vi "AlliGator Draw Phasor Plot UC.vi"(7 "# Ticks":i32=11, 8 "Error In":errorcluster, 11 "Phasor Plot Image  in":T2) -> (0 "Error Out":errorcluster, 1 "Font, Size & Style":T1, 2 "Phasor Plot Frame Reference Points":T3, 3 "Phasor Plot Image out":T2)   [LabVIEW 2021, in "AlliGator Phasor Plot.lvlib"]
doc: "Draws the UC in the Phasor Plot image."
uses:
  AlliGator Phasor Plot.lvlib
  <vilib>/vision/Image Controls.llb/IMAQ Image.ctl
  Phasor Ratio/AlliGator Phasor Plot Reference Points.ctl
  Phasor/Phasor SEPL Tick Data.ctl
  Phasor/Phasor (g, s).ctl
  Phasor Ratio/AlliGator Phasor Ratio.lvlib
  Utilities/Utilities.lvlib
  Math/Math.lvlib
  Settings/AlliGator Settings.lvlib
  Phasor/Phasor.lvlib
panel:
  # "see the AlliGator License on the block diagram (Ctrl+E or Window:Show Block Diagram)"
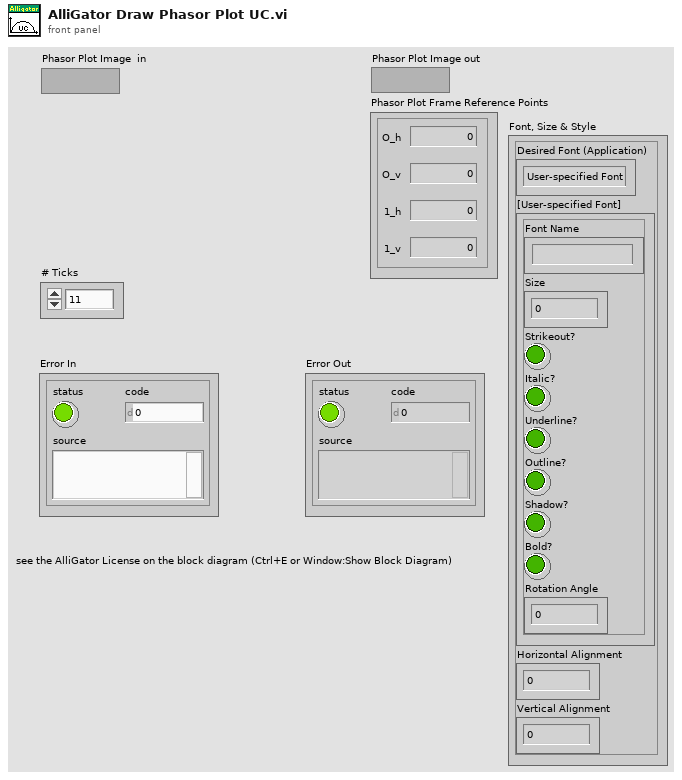
[diagram p1: front panel]
types:
  T1 = cluster{"Desired Font (Application)":enum16{"User-specified Font", "Application Font", "System Font", "Dialog Font"}, "[User-specified Font]":cluster{"Font Name":string, "Size":i16, "Strikeout?":bool, "Italic?":bool, "Underline?":bool, "Outline?":bool, "Shadow?":bool, "Bold?":bool, "Rotation Angle":dbl}, "Horizontal Alignment":i16, "Vertical Alignment":i16}
  T2 = typedef "IMAQ Image.ctl" = refnum<image>
  T3 = typedef "AlliGator Phasor Ratio.lvlib/AlliGator Phasor Plot Reference Points.ctl" = cluster{"O_h":dbl, "O_v":dbl, "1_h":dbl, "1_v":dbl}
  T4 = typedef "AlliGator Settings.lvlib/AlliGator Phasor Plot Graphics Options.ctl" = cluster{"UC Color":u32, "Show UC Tau Ticks":bool, "SEPL Color":u32, "Show SEPL Tau Ticks":bool, "Axes Color":u32, "Show (g,s) Ticks":bool, "Show UC":bool, "Show SEPL":bool, "Show Axes":bool, "Show UC Tau Labels":bool, "Show SEPL Tau Labels":bool, "Show (g,s) Labels":bool, "UC Label Size":i16, "UC Label Distance":dbl, "SEPL Label Size":i16, "SEPL Label Distance":dbl, "Axes Label Size":i16, "Axes Label Distance":dbl}
  T5 = typedef "AlliGator Phasor Plot.lvlib/AlliGator Phasor Plot Size.ctl" = cluster{"H":i32, "V":i32, "Margin":dbl}
  T6 = cluster{"UCl":dbl, "UCt":dbl, "UCr":dbl, "UCb":dbl}
  T7 = typedef "Phasor.lvlib/Phasor SEPL Tick Data.ctl" = cluster{"tau_i (ns)":dbl, "Tick start (g, s)":T8, "Tick (dg, ds)":T8, "long tick?":bool}
  T8 = typedef "Phasor.lvlib/Phasor (g, s).ctl" = cluster{"g":dbl, "s":dbl}
  T9 = cluster{"Phasor Plot x":dbl, "Phasor Plot y":dbl}
  T10 = typedef "Utilities.lvlib/For Loop Iteration Type.ctl" = enum16{"default", "first", "last", "out of range"}
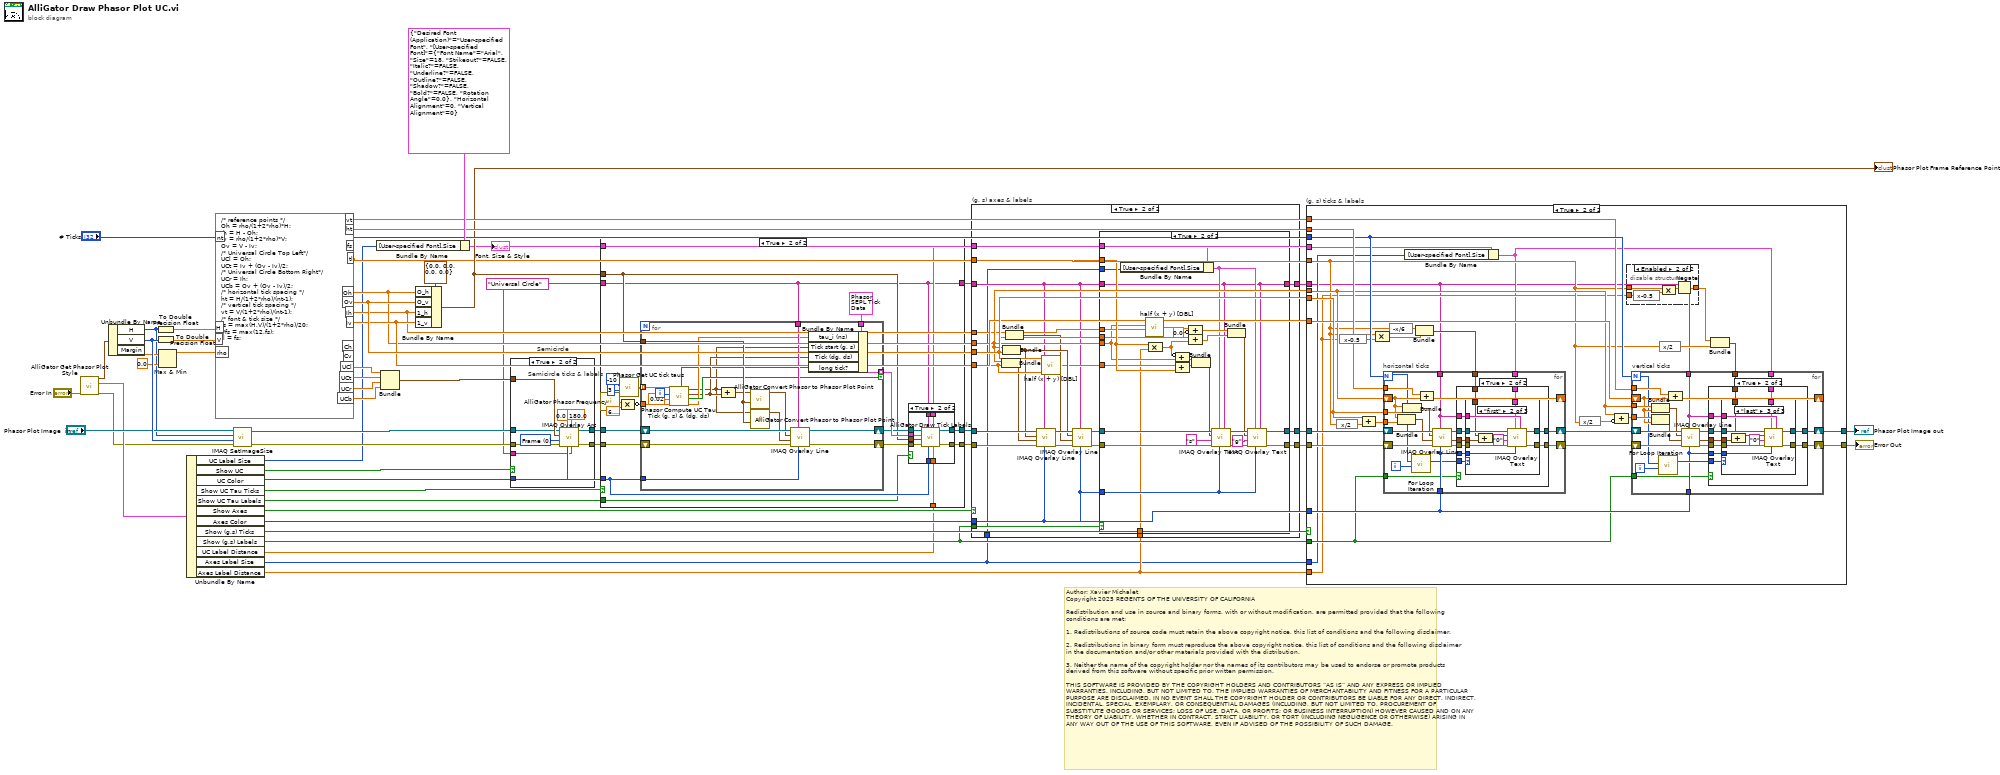
[diagram p0: block diagram]
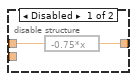
[diagram p7: hidden frame]
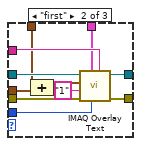
[diagram p10: hidden frame]
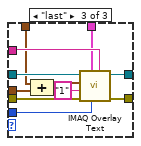
[diagram p13: hidden frame]
diagram:
  w13 = "Universal Circle" ("Group")
  # "Author: Xavier Michalet\nCopyright 2025 REGENTS OF THE UNIVERSITY OF CALIFORNIA\n\nRedistribution and use in source and binary forms, with or without modification, are permitted provided that the following conditions are met:\n\n1. Redistributions of source code must retain the above copyright notice, this list of conditions and the following disclaimer.\n\n2. Redistributions in binary form must reproduce the above copyright notice, this list of conditions and the following disclaimer in the documentation and/or other materials provided with the distribution.\n\n3. Neither the name of the copyright holder nor the names of its contributors may be used to endorse or promote products derived from this software without specific prior written permission.\n\nTHIS SOFTWARE IS PROVIDED BY THE COPYRIGHT HOLDERS AND CONTRIBUTORS “AS IS” AND ANY EXPRESS OR IMPLIED WARRANTIES, INCLUDING, BUT NOT LIMITED TO, THE IMPLIED WARRANTIES OF MERCHANTABILITY AND FITNESS FOR A PARTICULAR PURPOSE ARE DISCLAIMED. IN NO EVENT SHALL THE COPYRIGHT HOLDER OR CONTRIBUTORS BE LIABLE FOR ANY DIRECT, INDIRECT, INCIDENTAL, SPECIAL, EXEMPLARY, OR CONSEQUENTIAL DAMAGES (INCLUDING, BUT NOT LIMITED TO, PROCUREMENT OF SUBSTITUTE GOODS OR SERVICES; LOSS OF USE, DATA, OR PROFITS; OR BUSINESS INTERRUPTION) HOWEVER CAUSED AND ON ANY THEORY OF LIABILITY, WHETHER IN CONTRACT, STRICT LIABILITY, OR TORT (INCLUDING NEGLIGENCE OR OTHERWISE) ARISING IN ANY WAY OUT OF THE USE OF THIS SOFTWARE, EVEN IF ADVISED OF THE POSSIBILITY OF SUCH DAMAGE."
  n1 = call "AlliGator Get Phasor Plot Style.vi"("Error In"="Error In") -> ("Error Out"=w15:errorcluster, "Phasor Plot Graphics Options"=w18:T4, "Phasor Plot Size"=w17:T5)  [unwired: 8 in]
  n2 = Unbundle By Name(w17) -> ("H"=w8:i32, "V"=w45:i32, "Margin"=w37:dbl)
  n3 = To Double Precision Float(number=w8) -> (double precision float=w48:dbl)
  n4 = To Double Precision Float(number=w45) -> (double precision float=w47:dbl)
  n5 = Max & Min(x=w37, y=0.0) -> (max(x,y)=w35:dbl)  [unwired: 1 out]
  n6 = Unbundle By Name(w18) -> ("UC Label Size"=w6:i16, "Show UC"=w25:bool, "UC Color"=w23:u32, "Show UC Tau Ticks"=w24:bool, "Show UC Tau Labels"=w10:bool, "Show Axes"=w26:bool, "Axes Color"=w30:u32, "Show (g,s) Ticks"=w27:bool, "Show (g,s) Labels"=w11:bool, "UC Label Distance"=w5:dbl, "Axes Label Size"=w3:i16, "Axes Label Distance"=w4:dbl)
  n7 = formula code="/* reference points */\nOh = rho/(1+2*rho)*H;\nIh = H - Oh;\nIv = rho/(1+2*rho)*V;\nOv = V - Iv;\n/* Universal Circle Top Left*/\nUCl = Oh;\nUCt = Iv + (Ov - Iv)/2;\n/* Universal Circle Bottom Right*/\nUCr = Ih;\nUCb = Ov + (Ov - Iv)/2;\n/* horizontal tick spacing */\nht = H/(1+2*rho)/(nt-1);\n/* vertical tick spacing */\nvt = V/(1+2*rho)/(nt-1);\n/* font & tick size */\nfs = max(H,V)/(1+2*rho)/20;\n//fs = max(12,fs);\ntl = fs;"("H"=w48, "V"=w47, "rho"=w35, "nt"="# Ticks") -> ("Oh"=w32:dbl, "Ov"=w34:dbl, "Ih"=w31:dbl, "Iv"=w33:dbl, "UCl"=w51:dbl, "UCt"=w52:dbl, "UCr"=w50:dbl, "UCb"=w49:dbl, "ht"=w42:dbl, "vt"=w38:dbl, "tl"=w7:dbl)  [unwired: 3 out]
  n8 = call "IMAQ SetImageSize"("error in (no error)"=w15, "Y Resolution"=w45, "X Resolution"=w8, "Image"="Phasor Plot Image  in") -> ("error out"=w43:errorcluster, "Image Out"=w46:T2)  [unwired: 1 in]
  n9 = Bundle By Name(cluster=T1 {"Desired Font (Application)"=enum."User-specified Font", "[User-specified Font]"={"Font Name"="Arial", "Size"=18, "Strikeout?"=FALSE, "Italic?"=FALSE, "Underline?"=FALSE, "Outline?"=FALSE, "Shadow?"=FALSE, "Bold?"=FALSE, "Rotation Angle"=0.0}, "Horizontal Alignment"=0, "Vertical Alignment"=0} ("Font, Size & Style"), "[User-specified Font].Size"=w6) -> (w9:T1)
  "Font, Size & Style" <- w9
  n10 = Bundle("UCl"=w51, "UCt"=w52, "UCr"=w50, "UCb"=w49) -> (w14:T6)  [unwired: 1 in]
  n11 = Bundle By Name(cluster=T3 {"O_h"=0.0, "O_v"=0.0, "1_h"=0.0, "1_v"=0.0} ("Phasor Plot Reference Points"), "O_h"=w32, "O_v"=w34, "1_h"=w31, "1_v"=w33) -> (w12:T3)
  "Phasor Plot Frame Reference Points" <- w12
  n12 = case "Semicircle" shown="True" w25 {
    tunnel: w14 -> [_ w66]
    tunnel: w46 -> [w56 w65]
    tunnel: w43 -> [w55 w64]
    tunnel: w23 -> [_ w63]
    tunnel: [w56 w59] -> w22
    tunnel: [w55 w58] -> w21
    tunnel: w13 -> [_ w57]
    frame False {
    }
    frame True {
      w62 = u32 0 items=["Frame", "Fill"] ("Drawing Mode (Frame)")
      n13 = call "IMAQ Overlay Arc"("Group"=w57, "End Angle (degrees)"=180.0, "Color"=w63, "Start Angle (degrees)"=0.0, "error in (no error)"=w64, "Drawing Mode (Frame)"=w62, "Bounding Rectangle"=w66, "Image"=w65) -> ("error out"=w58:errorcluster, "Image Out"=w59:T2)  [unwired: 2 in]
    }
  }
  n14 = case "Semicircle ticks & labels" shown="True" w24 {
    tunnel: w23 -> [_ w76]
    tunnel: [w69 w81] -> w20
    tunnel: w22 -> [w69 w85]
    tunnel: [w68 w79] -> w19
    tunnel: w21 -> [w68 w84]
    tunnel: w13 -> [w67 w70]
    tunnel: w12 -> [_ w72]
    tunnel: w10 -> [_ w75]
    tunnel: w9 -> [_ w78]
    tunnel: w5 -> [_ w71]
    tunnel: [w67 w70] -> w2
    frame False {
    }
    frame True {
      n15 = call "AlliGator Phasor Frequency.vi"() -> ("Phasor Frequency"=w88:dbl[unit])
      n16 = call "Phasor Get UC tick taus.vi"("Log Tick Start (-10: 100 ps)"=-10, "# Decades (4: 10 ps - 900 ns)"=3) -> ("Array of taus"=w89:dbl[unit][])  [unwired: 6 in]
      n17 = Compound Arithmetic op=MULTIPLY(w88, 6.283185307179586) -> (invert w87:dbl[unit])
      n18 = for {
        tunnel: w89 -> [w122] mode=indexing
        tunnel: w87 -> [w120]
        tunnel: w72 -> [w119]
        shift-right: [w114] -> w82
        shift-left: w85 -> [w118]
        shift-right: [w113] -> w80
        shift-left: w84 -> [w115]
        tunnel: w70 -> [w112]
        tunnel: w76 -> [w111]
        tunnel: [w105] -> w83 mode=indexing if=w108
        tunnel: T7 {"tau_i (ns)"=0.0, "Tick start (g, s)"={"g"=0.0, "s"=0.0}, "Tick (dg, ds)"={"g"=0.0, "s"=0.0}, "long tick?"=FALSE} -> [w102]
        i -> [w121]
        n19 = call "Phasor Compute UC Tau Tick (g, s) & (dg, ds).vi"("1/2 pi f"=w120, "Tick Length (0.01)"=0.02, "Tick Index"=w121, "tau_i"=w122) -> ("tau_i (ns)"=w107:dbl, "label?"=w108:bool, "Tick (dg, ds)"=w106:T8, "Tick start (g, s)"=w103:T8, "long tick?"=w104:bool)  [unwired: 3 in]
        n20 = Compound Arithmetic op=ADD(w103, w106) -> (w109:T8)
        n21 = call "AlliGator Convert Phasor to Phasor Plot Point.vi"("Phasor Plot Reference Points"=w119, "Phasor"=w109) -> ("Phasor Plot Point"=w117:T9)  [unwired: 9 in]
        n22 = call "AlliGator Convert Phasor to Phasor Plot Point.vi"("Phasor Plot Reference Points"=w119, "Phasor"=w103) -> ("Phasor Plot Point"=w116:T9)  [unwired: 9 in]
        n23 = call "IMAQ Overlay Line"("Color"=w111, "Group"=w112, "error in (no error)"=w115, "End Point"=w116, "Start Point"=w117, "Image"=w118) -> ("error out"=w113:errorcluster, "Image Out"=w114:T2)  [unwired: 4 in]
        n24 = Bundle By Name(cluster=w102, "tau_i (ns)"=w107, "Tick start (g, s)"=w103, "Tick (dg, ds)"=w106, "long tick?"=w104) -> (w105:T7)
      }
      n25 = case shown="True" w75 {
        tunnel: w83 -> [_ w94]
        tunnel: w82 -> [w91 w101]
        tunnel: [w91 w100] -> w81
        tunnel: w80 -> [w90 w99]
        tunnel: [w90 w98] -> w79
        tunnel: w70 -> [_ w97]
        tunnel: w78 -> [_ w96]
        tunnel: w76 -> [_ w95]
        tunnel: w72 -> [_ w93]
        tunnel: w71 -> [_ w92]
        frame False {
        }
        frame True {
          n26 = call "AlliGator Draw Tick Labels.vi"("Label Distance (tick unit)"=w92, "Font, Size & Style"=w96, "Text Color"=w95, "Overlay Group"=w97, "error in (no error)"=w99, "Phasor Plot Reference Points"=w93, "Tick Label Data"=w94, "Refnum in"=w101) -> ("error out"=w98:errorcluster, "Refnum out"=w100:T2)  [unwired: 2 in]
        }
      }
    }
  }
  n27 = case "(g, s) axes & labels" shown="True" w26 {
    tunnel: w9 -> [_ w149]
    tunnel: w7 -> [_ w148]
    tunnel: w34 -> [_ w147]
    tunnel: w33 -> [_ w146]
    tunnel: w32 -> [_ w145]
    tunnel: w31 -> [_ w144]
    tunnel: w30 -> [_ w129]
    tunnel: w20 -> [w125 w143]
    tunnel: w19 -> [w124 w140]
    tunnel: [w125 w134] -> w29
    tunnel: [w124 w133] -> w28
    tunnel: w2 -> [w123 w131]
    tunnel: w11 -> [_ w130]
    tunnel: w3 -> [_ w128]
    tunnel: w4 -> [_ w127]
    tunnel: [w123 w126] -> w1
    frame False {
    }
    frame True {
      n28 = Bundle("Oh"=w145, "Iv"=w146) -> (w137:cluster{"Oh":dbl, "Iv":dbl})  [unwired: 1 in]
      n29 = Bundle("Oh"=w145, "Ov"=w147) -> (w136:cluster{"Oh":dbl, "Ov":dbl})  [unwired: 1 in]
      n30 = Bundle("Ih"=w144, "Ov"=w147) -> (w135:cluster{"Ih":dbl, "Ov":dbl})  [unwired: 1 in]
      n31 = call "IMAQ Overlay Line"("Color"=w129, "Group"=w131, "error in (no error)"=w140, "End Point"=w137, "Start Point"=w136, "Image"=w143) -> ("error out"=w141:errorcluster, "Image Out"=w142:T2)  [unwired: 4 in]
      n32 = call "half (x + y) [DBL].vi"("y"=w146, "x"=w147) -> ("(x+y)/2"=w132:dbl)  [unwired: 4 in]
      n33 = call "IMAQ Overlay Line"("Color"=w129, "Group"=w131, "error in (no error)"=w141, "End Point"=w135, "Start Point"=w136, "Image"=w142) -> ("error out"=w138:errorcluster, "Image Out"=w139:T2)  [unwired: 4 in]
      n34 = case shown="True" w130 {
        tunnel: w149 -> [_ w180]
        tunnel: w148 -> [_ w179]
        tunnel: w147 -> [_ w178]
        tunnel: w145 -> [_ w155]
        tunnel: w144 -> [_ w177]
        tunnel: w139 -> [w152 w176]
        tunnel: w138 -> [w151 w175]
        tunnel: [w152 w164] -> w134
        tunnel: [w151 w163] -> w133
        tunnel: w132 -> [_ w162]
        tunnel: w131 -> [w150 w153]
        tunnel: w129 -> [_ w158]
        tunnel: w128 -> [_ w156]
        tunnel: w127 -> [_ w154]
        tunnel: [w150 w153] -> w126
        frame False {
        }
        frame True {
          n35 = Bundle By Name(cluster=w180, "[User-specified Font].Size"=w156) -> (w157:T1)
          n36 = call "half (x + y) [DBL].vi"("y"=w177, "x"=w155) -> ("(x+y)/2"=w161:dbl)  [unwired: 4 in]
          n37 = Compound Arithmetic op=MULTIPLY(w179, w154) -> (w159:dbl)
          n38 = Compound Arithmetic op=ADD(invert w159, w155) -> (w170:dbl)
          n39 = Compound Arithmetic op=ADD(w162, w179) -> (w169:dbl)
          n40 = Compound Arithmetic op=ADD(w161, invert 0.0 ("value")) -> (w167:dbl)
          n41 = Compound Arithmetic op=ADD(w178, w159) -> (w166:dbl)
          n42 = Bundle(w170, w169) -> (w168:cluster{dbl, dbl})  [unwired: 1 in]
          n43 = call "IMAQ Overlay Text"("Group"=w153, "Text Color (black)"=w158, "Font, Size & Style"=w157, "error in (no error)"=w175, "String"="s", "Origin"=w168, "Image"=w176) -> ("error out"=w174:errorcluster, "Image Out"=w173:T2)  [unwired: 3 in]
          n44 = Bundle(w167, w166) -> (w165:cluster{dbl, dbl})  [unwired: 1 in]
          n45 = call "IMAQ Overlay Text"("Group"=w153, "Text Color (black)"=w158, "Font, Size & Style"=w157, "error in (no error)"=w174, "String"="g", "Origin"=w165, "Image"=w173) -> ("error out"=w163:errorcluster, "Image Out"=w164:T2)  [unwired: 3 in]
        }
      }
    }
  }
  n46 = case "(g, s) ticks & labels" shown="True" w27 {
    tunnel: w42 -> [_ w213]
    tunnel: [w182 w212] -> w41
    tunnel: [w181 w211] -> w40
    tunnel: "# Ticks" -> [_ w210]
    tunnel: w38 -> [_ w209]
    tunnel: w9 -> [_ w186]
    tunnel: w7 -> [_ w191]
    tunnel: w34 -> [_ w208]
    tunnel: w33 -> [_ w207]
    tunnel: w32 -> [_ w206]
    tunnel: w30 -> [_ w205]
    tunnel: w29 -> [w182 w204]
    tunnel: w28 -> [w181 w203]
    tunnel: w11 -> [_ w190]
    tunnel: w4 -> [_ w188]
    tunnel: w3 -> [_ w185]
    tunnel: w1 -> [_ w183]
    frame False {
    }
    frame True {
      n47 = expression code="x/2"(w191) -> (w201:dbl)
      n48 = expression code="x-0.5"(w188) -> (w184:dbl)
      n49 = Compound Arithmetic op=ADD(w208, w201) -> (w202:dbl)
      n50 = Compound Arithmetic op=MULTIPLY(w191, w184) -> (w189:dbl)
      n51 = expression code="-x/6"(w191) -> (w195:dbl)
      n52 = Bundle By Name(cluster=w186, "[User-specified Font].Size"=w185) -> (w187:T1)
      n53 = Bundle("tl"=w195, w189) -> (w196:cluster{"tl":dbl, dbl})  [unwired: 1 in]
      n54 = for "horizontal ticks" {
        N: w210 -> [w283]
        shift-right: [w288] -> w200
        shift-left: w204 -> [w298]
        shift-right: [w287] -> w199
        shift-left: w203 -> [w297]
        shift-right: [w294] -> _
        shift-left: w206 -> [w292]
        tunnel: w205 -> [w285]
        tunnel: w213 -> [w293]
        tunnel: w202 -> [w291]
        tunnel: w183 -> [w286]
        tunnel: w208 -> [w296]
        tunnel: w187 -> [w281]
        tunnel: w196 -> [w279]
        tunnel: w190 -> [w278]
        i -> [w284]
        n55 = Bundle("Oh"=w292, w291) -> (w280:cluster{"Oh":dbl, dbl})  [unwired: 1 in]
        n56 = Bundle("Oh"=w292, "Ov"=w296) -> (w295:cluster{"Oh":dbl, "Ov":dbl})  [unwired: 1 in]
        n57 = call "For Loop Iteration.vi"("i"=w284, "N"=w283) -> ("Iteration"=w282:T10)  [unwired: 8 in, 1 out]
        n58 = Compound Arithmetic op=ADD(w293, w292) -> (w294:dbl)
        n59 = call "IMAQ Overlay Line"("Color"=w285, "Group"=w286, "error in (no error)"=w297, "End Point"=w280, "Start Point"=w295, "Image"=w298) -> ("error out"=w289:errorcluster, "Image Out"=w290:T2)  [unwired: 4 in]
        n60 = case shown="True" w278 {
          tunnel: w290 -> [w300 w310]
          tunnel: w289 -> [w299 w309]
          tunnel: [w300 w308] -> w288
          tunnel: [w299 w307] -> w287
          tunnel: w286 -> [_ w306]
          tunnel: w285 -> [_ w305]
          tunnel: w282 -> [_ w304]
          tunnel: w281 -> [_ w303]
          tunnel: w280 -> [_ w302]
          tunnel: w279 -> [_ w301]
          frame False {
          }
          frame True {
            n61 = case shown="\"first\"" w304 {
              tunnel: w310 -> [w312 w323 w334]
              tunnel: w309 -> [w311 w322 w333]
              tunnel: [w312 w321 w332] -> w308
              tunnel: [w311 w320 w331] -> w307
              tunnel: w306 -> [_ w319 w330]
              tunnel: w305 -> [_ w318 w329]
              tunnel: w303 -> [_ w313 w327]
              tunnel: w302 -> [_ w316 w326]
              tunnel: w301 -> [_ w315 w325]
              frame "default", Default {
              }
              frame "first" {
                n62 = Compound Arithmetic op=ADD(w315, w316) -> (w314:cluster{dbl, dbl})
                n63 = call "IMAQ Overlay Text"("Group"=w319, "Text Color (black)"=w318, "Font, Size & Style"=w313, "error in (no error)"=w322, "String"="0", "Origin"=w314, "Image"=w323) -> ("error out"=w320:errorcluster, "Image Out"=w321:T2)  [unwired: 3 in]
              }
              frame "last" {
                n64 = Compound Arithmetic op=ADD(w325, w326) -> (w324:cluster{dbl, dbl})
                n65 = call "IMAQ Overlay Text"("Group"=w330, "Text Color (black)"=w329, "Font, Size & Style"=w327, "error in (no error)"=w333, "String"="1", "Origin"=w324, "Image"=w334) -> ("error out"=w331:errorcluster, "Image Out"=w332:T2)  [unwired: 3 in]
              }
            }
          }
        }
      }
      n66 = expression code="x/2"(w191) -> (w198:dbl)
      n67 = Compound Arithmetic op=ADD(w206, invert w198) -> (w197:dbl)
      n68 = disable-structure shown="Enabled" {
        disable-tunnel: [w215 w218] -> w193
        disable-tunnel: w191 -> [w214 w220]
        disable-tunnel: w188 -> [_ w217]
        frame Disabled {
          n69 = expression code="-0.75*x"(w214) -> (w215:dbl)
        }
        frame Enabled {
          n70 = expression code="x-0.5"(w217) -> (w216:dbl)
          n71 = Compound Arithmetic op=MULTIPLY(w220, w216) -> (w219:dbl)
          n72 = Negate(x=w219) -> (-x=w218:dbl)
        }
      }
      n73 = expression code="x/2"(w191) -> (w192:dbl)
      n74 = Bundle(w193, "tl"=w192) -> (w194:cluster{dbl, "tl":dbl})  [unwired: 1 in]
      n75 = for "vertical ticks" {
        N: w210 -> [w228]
        shift-right: [w231] -> w212
        shift-left: w200 -> [w241]
        shift-right: [w230] -> w211
        shift-left: w199 -> [w240]
        shift-right: [w239] -> _
        shift-left: w207 -> [w234]
        tunnel: w205 -> [w224]
        tunnel: w209 -> [w238]
        tunnel: w183 -> [w226]
        tunnel: w206 -> [w237]
        tunnel: w197 -> [w236]
        tunnel: w187 -> [w225]
        tunnel: w194 -> [w222]
        tunnel: w190 -> [w221]
        i -> [w229]
        n76 = Bundle("Oh"=w237, "Iv"=w234) -> (w235:cluster{"Oh":dbl, "Iv":dbl})  [unwired: 1 in]
        n77 = Bundle(w236, "Iv"=w234) -> (w223:cluster{dbl, "Iv":dbl})  [unwired: 1 in]
        n78 = call "For Loop Iteration.vi"("i"=w229, "N"=w228) -> ("Iteration"=w227:T10)  [unwired: 8 in, 1 out]
        n79 = Compound Arithmetic op=ADD(w238, w234) -> (w239:dbl)
        n80 = call "IMAQ Overlay Line"("Color"=w224, "Group"=w226, "error in (no error)"=w240, "End Point"=w223, "Start Point"=w235, "Image"=w241) -> ("error out"=w232:errorcluster, "Image Out"=w233:T2)  [unwired: 4 in]
        n81 = case shown="True" w221 {
          tunnel: w233 -> [w243 w253]
          tunnel: w232 -> [w242 w252]
          tunnel: [w243 w251] -> w231
          tunnel: [w242 w250] -> w230
          tunnel: w227 -> [_ w249]
          tunnel: w226 -> [_ w248]
          tunnel: w225 -> [_ w247]
          tunnel: w224 -> [_ w246]
          tunnel: w223 -> [_ w245]
          tunnel: w222 -> [_ w244]
          frame False {
          }
          frame True {
            n82 = case shown="\"last\"" w249 {
              tunnel: w253 -> [w255 w266 w277]
              tunnel: w252 -> [w254 w265 w276]
              tunnel: [w255 w264 w275] -> w251
              tunnel: [w254 w263 w274] -> w250
              tunnel: w248 -> [_ w262 w273]
              tunnel: w246 -> [_ w261 w272]
              tunnel: w247 -> [_ w259 w267]
              tunnel: w245 -> [_ w258 w270]
              tunnel: w244 -> [_ w257 w269]
              frame "default", Default {
              }
              frame "first" {
                n83 = Compound Arithmetic op=ADD(w257, w258) -> (w256:cluster{dbl, dbl})
                n84 = call "IMAQ Overlay Text"("Group"=w262, "Text Color (black)"=w261, "Font, Size & Style"=w259, "error in (no error)"=w265, "String"="1", "Origin"=w256, "Image"=w266) -> ("error out"=w263:errorcluster, "Image Out"=w264:T2)  [unwired: 3 in]
              }
              frame "last" {
                n85 = Compound Arithmetic op=ADD(w269, w270) -> (w268:cluster{dbl, dbl})
                n86 = call "IMAQ Overlay Text"("Group"=w273, "Text Color (black)"=w272, "Font, Size & Style"=w267, "error in (no error)"=w276, "String"="0", "Origin"=w268, "Image"=w277) -> ("error out"=w274:errorcluster, "Image Out"=w275:T2)  [unwired: 3 in]
              }
            }
          }
        }
      }
    }
  }
  "Phasor Plot Image out" <- w41
  "Error Out" <- w40
